vi "剖面数据发送帧.vi"(11 "用户地址":string) -> (3 "数据帧":string[](array[string]))   [LabVIEW 2016, in "环境动力监测库.lvlib" / "NMEA.lvlib"]
uses:
  NMEA.lvlib
panel:
  out "数据帧长度":i32[](array[numeric])
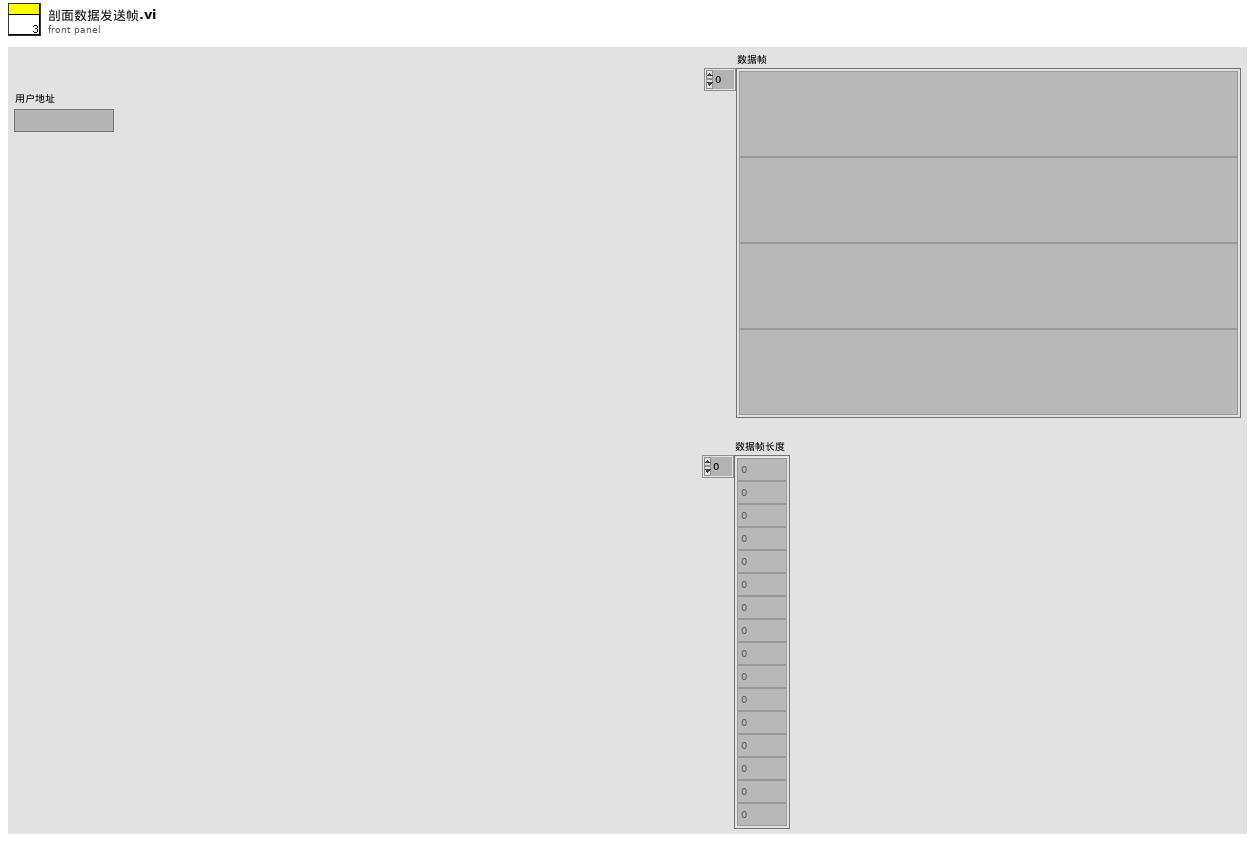
[diagram p1: front panel]
types:
  T1 = cluster{"污染物":u16, "检测值":dbl, "标识":u16, "标样浓度":dbl, "跨度值":dbl}[][]
  T2 = cluster{"数据类别":u16, "时间戳":timestamp, "数组":cluster{"污染物":u16, "检测值":dbl, "标识":u16, "标样浓度":dbl, "跨度值":dbl}[]}
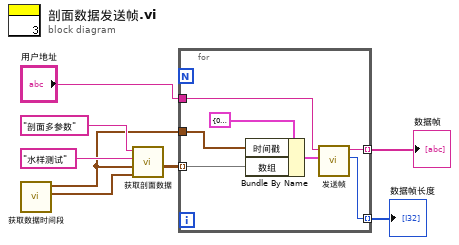
[diagram p0: block diagram]
diagram:
  n1 = call "获取数据时间段.vi"() -> ("end time"=w2:timestamp, "start time"=w1:timestamp)  [unwired: 10 in]
  n2 = call "获取剖面数据.vi"("end time"=w2, "start time"=w1, "测量模式"="水样测试", "table"="剖面多参数") -> ("数组"=w6:T1)  [unwired: 5 in, 2 out]
  n3 = for {
    tunnel: w6 -> [w14] mode=indexing
    tunnel: w1 -> [w13]
    tunnel: "用户地址" -> [w11]
    tunnel: [w10] -> w4 mode=indexing
    tunnel: [w9] -> w3 mode=indexing
    n4 = Bundle By Name(cluster=T2 {"数据类别"=0, "时间戳"=timestamp(0 s since 1904-01-01), "数组"=[]} ("data"), "时间戳"=w13, "数组"=w14) -> (w12:T2)
    n5 = call "发送帧.vi"("data"=w12, "用户地址"=w11) -> ("报文长度"=w9:i32, "字符串"=w10:string)  [unwired: 8 in]
  }
  "数据帧" <- w4
  "数据帧长度" <- w3
